vi "Start Test Selection (SubVI).vi"(8 "error in (no error)":errorcluster, 9 "TestArrayIn":string[](array[string])) -> (1 "AutoOut":bool, 2 "TestArrayOut":string[](array[string]))   [LabVIEW 2017]
panel:
  in  "Cancel":bool
  in  "Next Button":bool
  in  "Auto":bool
  in  "Listbox":i32[](listbox)
  # "Use Ctrl key to select many."
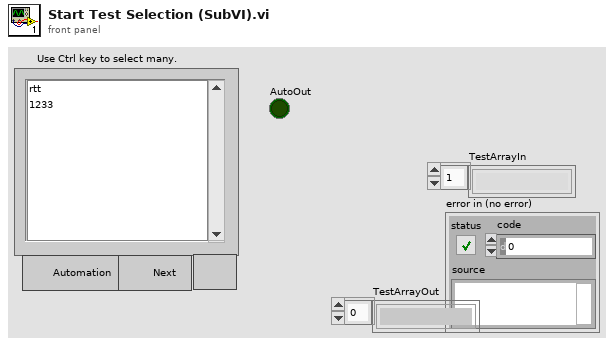
[diagram p1: front panel]
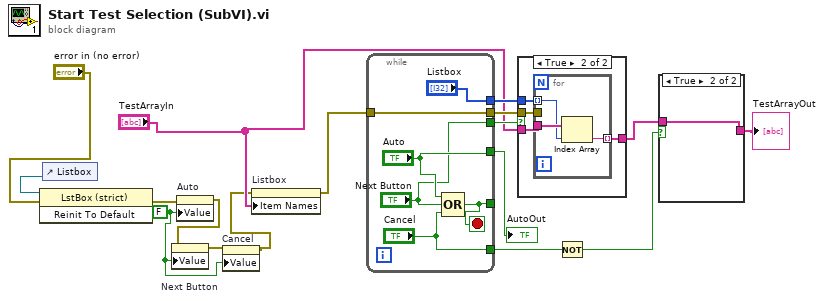
[diagram p0: block diagram]
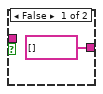
[diagram p2: hidden frame]
diagram:
  w4 = FALSE ("Auto")
  n1 = control-ref of="Listbox"() -> (w3:refnum<vi>)
  n2 = invoke class="LstBox (strict)" method="Reinit To Default"(reference=w3, error in="error in (no error)") -> (error out=w1:errorcluster)  [unwired: 1 in, 2 out]
  n3 = property on="Auto" class="Bool (strict)"(error in=w1, "Value"=w4) -> (error out=w14:errorcluster)  [unwired: 1 in, 1 out]
  n4 = property on="Next Button" class="Bool (strict)"(error in=w14, "Value"=w4) -> (error out=w5:errorcluster)  [unwired: 1 in, 1 out]
  n5 = property on="Cancel" class="Bool (strict)"(error in=w5, "Value"=w4) -> (error out=w6:errorcluster)  [unwired: 1 in, 1 out]
  n6 = property on="Listbox" class="LstBox (strict)"(error in=w6, "Item Names"="TestArrayIn") -> (error out=w16:errorcluster)  [unwired: 1 in, 1 out]
  n7 = while {
    tunnel: ["Listbox"] -> w17
    tunnel: w16 -> [w22]
    tunnel: [w22] -> w15
    tunnel: ["Next Button"] -> w13
    tunnel: ["Auto"] -> w12
    tunnel: [w19] -> _
    tunnel: ["Cancel"] -> w8
    stop <- w19 stop-if-true
    n8 = Compound Arithmetic op=OR("Auto", "Next Button", "Cancel") -> (w19:bool)
  }
  "AutoOut" <- w12
  n9 = case shown="True" w13 {
    tunnel: w17 -> [_ w28]
    tunnel: "TestArrayIn" -> [w24 w27]
    tunnel: w15 -> [_ w26]
    tunnel: [w24 w25] -> w10
    frame False {
    }
    frame True {
      n10 = for {
        tunnel: w28 -> [w29] mode=indexing
        tunnel: [w30] -> w25 mode=indexing
        tunnel: w27 -> [w31]
        tunnel: w26 -> [_]
        n11 = Index Array(array=w31, index=w29) -> (element=w30:string)
      }
    }
  }
  n12 = Not(x=w8) -> (.not. x?=w7:bool)
  n13 = case shown="True" w7 {
    tunnel: [string[] [] ("TestArrayIn") w33] -> w9
    tunnel: w10 -> [_ w33]
    frame False {
    }
    frame True {
    }
  }
  "TestArrayOut" <- w9
